vi "MeasurementServer_Stop.vi"(0 "Server Information":T2, 1 "Event Registration Refnum":refnum<event-registration>, 3 "error in (no error)":errorcluster) -> (10 "error out":errorcluster)   [LabVIEW 2019, in "labview-grpc-measurement-server.lvlib"]
uses:
  labview-grpc-measurement-server.lvlib
  MeasurementServer_InvokeEventData.ctl
  MeasurementServer_gRPCid.ctl
  home/lvuser/liblabview_measurement_server.so
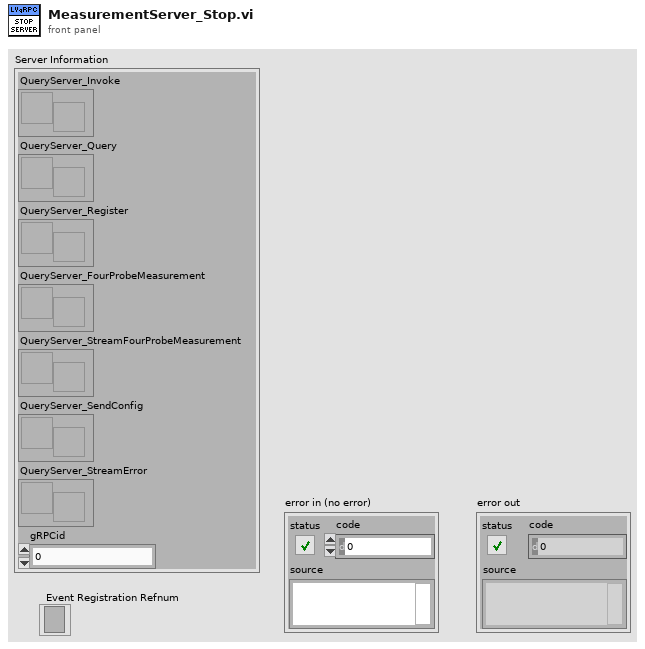
[diagram p1: front panel]
types:
  T1 = typedef "labview-grpc-measurement-server.lvlib/MeasurementServer_gRPCid.ctl" = u64
  T2 = cluster{"QueryServer_Invoke":refnum<user-event>, "QueryServer_Query":refnum<user-event>, "QueryServer_Register":refnum<user-event>, "QueryServer_FourProbeMeasurement":refnum<user-event>, "QueryServer_StreamFourProbeMeasurement":refnum<user-event>, "QueryServer_SendConfig":refnum<user-event>, "QueryServer_StreamError":refnum<user-event>, "gRPCid":T1}
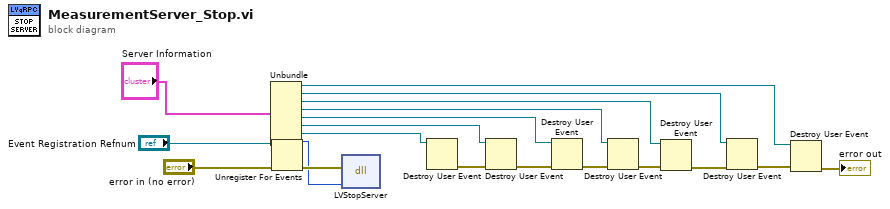
[diagram p0: block diagram]
diagram:
  n1 = Unbundle("Server Information") -> ("QueryServer_Invoke"=w12:refnum<user-event>, "QueryServer_Query"=w13:refnum<user-event>, "QueryServer_Register"=w14:refnum<user-event>, "QueryServer_FourProbeMeasurement"=w10:refnum<user-event>, "QueryServer_StreamFourProbeMeasurement"=w8:refnum<user-event>, "QueryServer_SendConfig"=w6:refnum<user-event>, "QueryServer_StreamError"=w1:refnum<user-event>, "gRPCid"=w3:T1)
  n2 = Unregister For Events(event registration refnum="Event Registration Refnum", error in="error in (no error)") -> (error out=w19:errorcluster)
  n3 = dll-call lib="home/lvuser/liblabview_measurement_server.so" fn="LVStopServer"(error in=w19, "server"=w3) -> ()  [unwired: 4 in, 2 out]
  n4 = Destroy User Event(user event=w1) -> (error out=w2:errorcluster)  [unwired: 1 in]
  n5 = Destroy User Event(user event=w6, error in=w2) -> (error out=w7:errorcluster)
  n6 = Destroy User Event(user event=w8, error in=w7) -> (error out=w9:errorcluster)
  n7 = Destroy User Event(user event=w10, error in=w9) -> (error out=w11:errorcluster)
  n8 = Destroy User Event(user event=w14, error in=w11) -> (error out=w17:errorcluster)
  n9 = Destroy User Event(user event=w13, error in=w17) -> (error out=w16:errorcluster)
  n10 = Destroy User Event(user event=w12, error in=w16) -> (error out=→"error out":errorcluster)
